vi "TelegramBOT_MainRPI.vi"() -> ()   [LabVIEW 2019]
uses:
  <vilib>/MakerHub/LINX/Private/Type Defs/LINX Ref.ctl
  <vilib>/MakerHub/LINX/Private/Type Defs/Platform.ctl
  <vilib>/MakerHub/LINX/Private/Type Defs/Interface.ctl
  <vilib>/MakerHub/LINX/Private/Device/Type Defs/LINX Device Config.ctl
  <vilib>/MakerHub/LINX/Private/Device/Type Defs/TCP Config.ctl
  <vilib>/MakerHub/LINX/Private/Device/Type Defs/Channels.ctl
  Demo 2 Sensor_SHT21/SHT21_class/SHT21.lvclass
  TelegramBOT_class/SendMsgType.ctl
  TelegramBOT_class/KeyboardMarkup.ctl
  <vilib>/MakerHub/LINX/Public/Peripherals/Digital/Digital Write 1 Chan.vi
  <vilib>/MakerHub/LINX/Public/Peripherals/Digital/Digital Write N Chans.vi
  <vilib>/MakerHub/LINX/Private/Local IO/LinxDigitalWrite.vi
  <vilib>/MakerHub/LINX/Public/Utilities/Check Channel.vi
  <vilib>/MakerHub/LINX/Private/Local IO/Handle Errors.vi
  <vilib>/MakerHub/LINX/Public/Utilities/Open Local.vi
  <vilib>/MakerHub/LINX/Private/Utilties/Generate Error.vi
  TelegramBOT_class/TelegramBOT.lvclass
  <vilib>/MakerHub/LINX/LMH-LINX.lvlib
  <vilib>/MakerHub/LINX/Private/Device/Device.lvlib
panel:
  out "From":string
  out "Message":string
  out "Message counter":i32
  in  "Stop":bool
  out "error out":errorcluster
  out "Connection":bool
  # "Demo live at our booth"
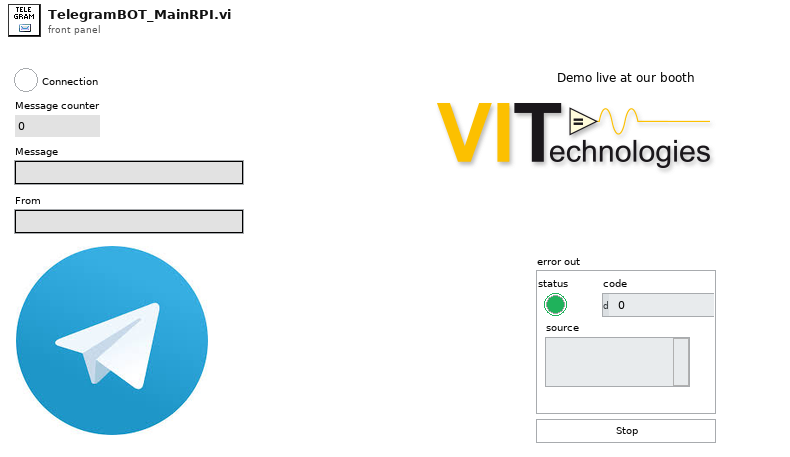
[diagram p1: front panel]
types:
  T1 = typedef "LMH-LINX.lvlib/LINX Ref.ctl" = cluster{"IO":T2, "Interface":T3, "LINX Device Config":T4}
  T2 = typedef "LMH-LINX.lvlib/Platform.ctl" = enum16{"Remote", "Local"}
  T3 = typedef "LMH-LINX.lvlib/Interface.ctl" = enum16{"Serial", "TCP"}
  T4 = typedef "LMH-LINX.lvlib/Device.lvlib/LINX Device Config.ctl" = cluster{"Interface":T3, "COM Port":refnum<visa-resource-name>, "TCP Configuration":T5, "Device Family":u8, "Device ID":u8, "Device Name":string, "TCP Ref":refnum<k5>, "Channels":T6}
  T5 = typedef "LMH-LINX.lvlib/Device.lvlib/TCP Config.ctl" = cluster{"IP Address":string, "Port":u16}
  T6 = typedef "LMH-LINX.lvlib/Channels.ctl" = cluster{"DI":u8[], "DO":u8[], "AI":u8[], "AO":u8[], "PWM":u8[], "QE":u8[], "UART":u8[], "I2C 2":u8[], "SPI":u8[], "CAN":u8[], "Servo":u8[], "AI Ref (V)":dbl, "AI Resolution (Bits)":u8, "AO Ref (V)":dbl, "AO Resolution (Bits)":u8}
  T7 = cluster{"LINX":T1, "SHT21":refnum<class "SHT21.lvclass">}
  T8 = typedef "TelegramBOT.lvclass/KeyboardMarkup.ctl" = cluster{"keyboard":cluster{"text":string, "req_loc":bool}[][], "resize_keyboard":bool, "one_time_keyboard":bool, "selective":bool}
  T9 = typedef "TelegramBOT.lvclass/SendMsgType.ctl" = enum16{"Text", "ReplyKeyboardMarkup", "ReplyKeyboardRemove"}
  T10 = typedef "TelegramBOT.lvclass/MessageCluster.ctl" = cluster{"update_id":u32, "from":string, "text":string, "date":timestamp, "chat_id":i32, "type":string, "reply_to_message.text":string, "message_id":u32}
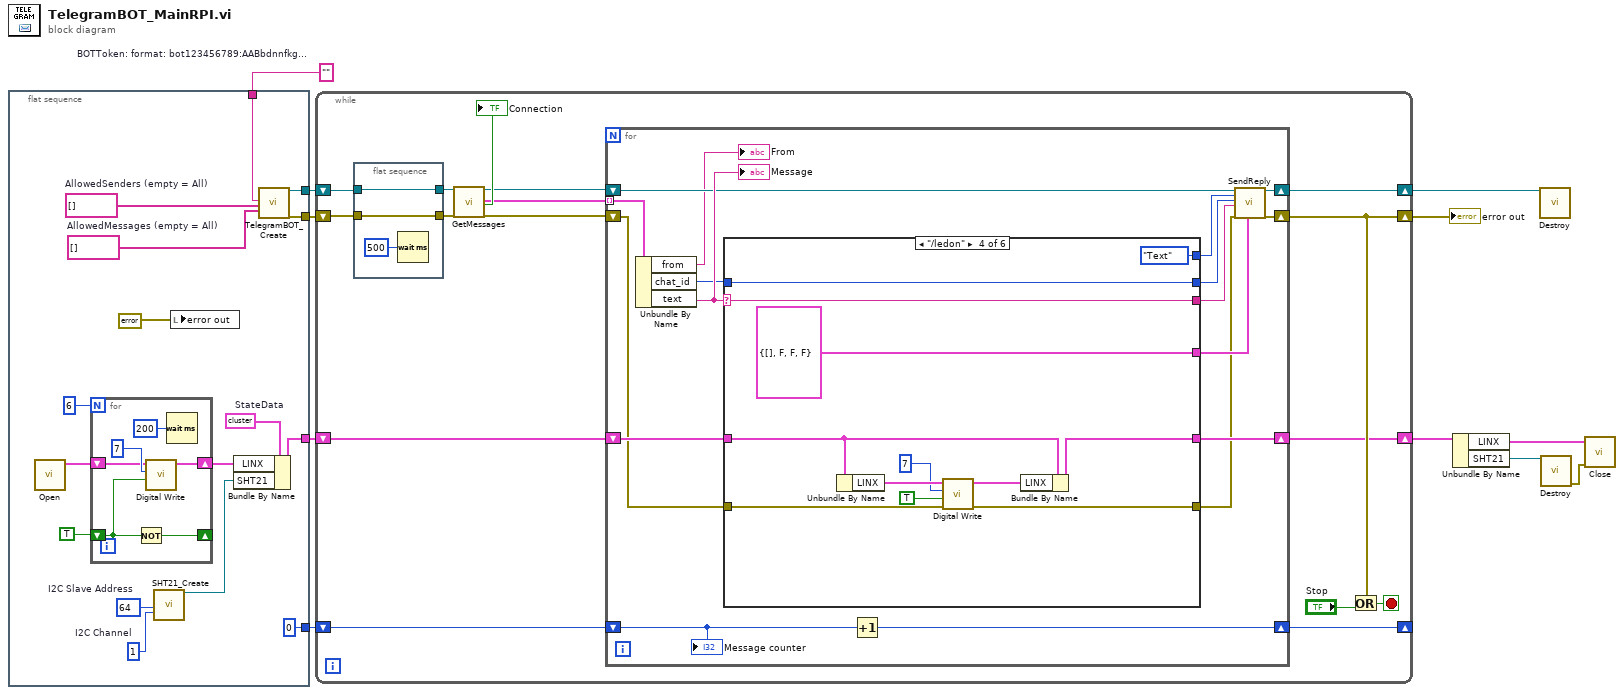
[diagram p0: block diagram]
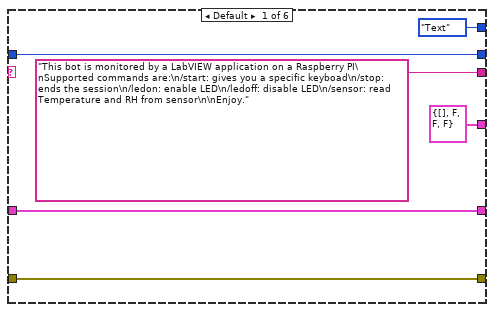
[diagram p2: hidden frame]
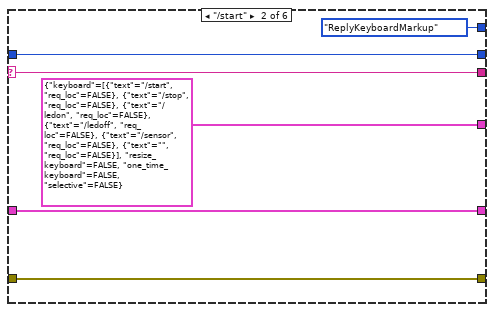
[diagram p3: hidden frame]
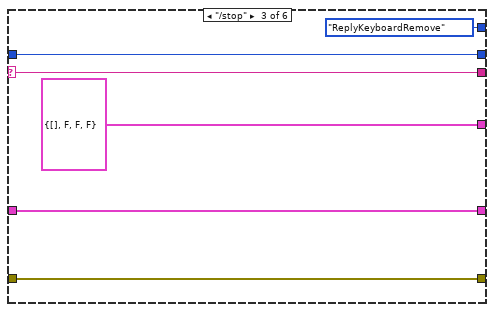
[diagram p4: hidden frame]
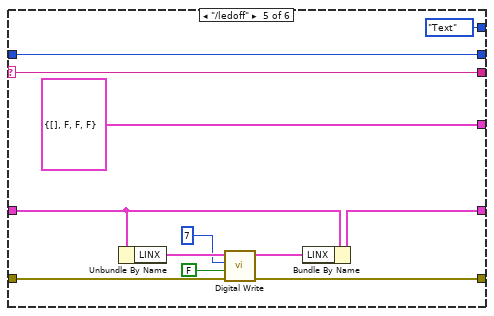
[diagram p5: hidden frame]
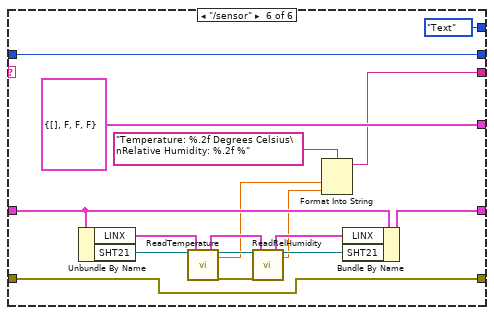
[diagram p6: hidden frame]
diagram:
  w7 = ""  # BOTToken: format: bot123456789:AABbdnnfkg...
  n1 = flat-sequence {
    tunnel: [w27] -> w11
    tunnel: [w26] -> w10
    tunnel: [0] -> w8
    tunnel: w7 -> [w24]
    tunnel: [w18] -> w1
    frame #0 {
      w20 = u8 1  # I2C Channel
      w21 = u8 64  # I2C Slave Address
      w19 = T7 {"LINX"={"IO"=enum."Remote", "Interface"=enum."Serial", "LINX Device Config"={"Interface"=enum."Serial", "COM Port"="COM13", "TCP Configuration"={"IP Address"="", "Port"=0}, "Device Family"=1, "Device ID"=1, "Device Name"="myRIO-1900", "TCP Ref"=refnum, "Channels"={"DI"=[0, 1, 2, 3, 4, 5, 6, 7, 8, 9, 10, 11, 12, 13, 14, 15, 16, 17, 18, 19, 20, 21, 22, 23, 24, 25, 26, 27, 28, 29, 30, 31, 32, 33, 34, 35, 36, 37, 38, 39, 40, 41, 42, 43, 44, 45, 46], "DO"=[0, 1, 2, 3, 4, 5, 6, 7, 8, 9, 10, 11, 12, 13, 14, 15, 16, 17, 18, 19, 20, 21, 22, 23, 24, 25, 26, 27, 28, 29, 30, 31, 32, 33, 34, 35, 36, 37, 38, 39, 40, 41, 42, 43, 44, 45, 46], "AI"=[0, 1, 2, 3, 4, 5, 6, 7, 8, 9, 10, 11], "AO"=[], "PWM"=[3, 5, 6, 9, 10], "QE"=[], "UART"=[0, 1], "I2C 2"=[0], "SPI"=[0], "CAN"=[], "Servo"=[], "AI Ref (V)"=0.0, "AI Resolution (Bits)"=0, "AO Ref (V)"=0.0, "AO Resolution (Bits)"=0}}}, "SHT21"=refnum}  # StateData
      w22 = string[] []  # AllowedMessages (empty = All)
      w23 = string[] []  # AllowedSenders (empty = All)
      n2 = call-poly <vilib>:"Open.vi"() -> ("LINX Resource"=w15:T1)  [unwired: 9 in, 2 out]
      n3 = for {
        N: 6 -> [_]
        shift-right: [w31] -> w14
        shift-left: w15 -> [w32]
        shift-right: [w30] -> _
        shift-left: TRUE ("Output Value") -> [w29]
        n4 = Not(x=w29) -> (.not. x?=w30:bool)
        n5 = call-poly <vilib>:"Digital Write.vi"("Output Value"=w29, "DO Channel"=u8 7, "LINX Resource"=w32) -> ("LINX Resource"=w31:T1)  [unwired: 7 in, 1 out]
        n6 = Wait (ms)(milliseconds to wait=u32 200) -> ()  [unwired: 1 out]
      }
      n7 = call "SHT21_Create.vi"("I2C Slave Address (0)"=w21, "I2C Channel (0)"=w20) -> ("reference out"=w17:refnum<class "SHT21.lvclass">)  [unwired: 16 in, 1 out]
      n8 = local write "error out"(errorcluster {"status"=FALSE, "code"=0, "source"=""} ("error out")) -> ()
      n9 = Bundle By Name(cluster=w19, "LINX"=w14, "SHT21"=w17) -> (w18:T7)
      n10 = call "TelegramBOT_Create.vi"("BOTToken(bot<token>)"=w24, "AllowedSenders (empty = All)"=w23, "AllowedMessages (empty = All)"=w22) -> ("reference out"=w27:refnum<class "TelegramBOT.lvclass">, "error out"=w26:errorcluster)  [unwired: 15 in]
    }
  }
  n11 = while {
    shift-right: [w34] -> w5
    shift-left: w1 -> [w35]
    shift-right: [w38] -> w6
    shift-left: w10 -> [w44]
    shift-right: [w42] -> w9
    shift-left: w11 -> [w45]
    shift-right: [w36] -> _
    shift-left: w8 -> [w37]
    stop <- w48 stop-if-true
    n12 = flat-sequence {
      tunnel: [w128] -> w46
      tunnel: w45 -> [w128]
      tunnel: [w127] -> w47
      tunnel: w44 -> [w127]
      frame #0 {
        n13 = Wait (ms)(milliseconds to wait=u32 500) -> ()  [unwired: 1 out]
      }
    }
    n14 = call-dynamic "GetMessages.vi"("reference in"=w46, "error in (no error)"=w47) -> ("reference out"=w41:refnum<class "TelegramBOT.lvclass">, "Messages"=w40:T10[], "Connection"=→"Connection":bool, "error out"=w39:errorcluster)  [unwired: 13 in, 1 out]
    n15 = for {
      shift-right: [w62] -> w42
      shift-left: w41 -> [w63]
      shift-right: [w61] -> w38
      shift-left: w39 -> [w51]
      tunnel: w40 -> [w66] mode=indexing
      shift-right: [w52] -> w34
      shift-left: w35 -> [w54]
      shift-right: [w55] -> w36
      shift-left: w37 -> [w56]
      n16 = Unbundle By Name(w66) -> ("from"=→"From":string, "chat_id"=w64:i32, "text"=w65:string)
      "Message" <- w65
      n17 = case shown="\"/ledon\"" w65 {
        selector: w65 -> [_ w78 w84 w96 w108 _]
        tunnel: w64 -> [w72 w77 w83 w95 w107 w125]
        tunnel: ["This bot is monitored by a LabVIEW application on a Raspberry PI\nSupported commands are:\n/start: gives you a specific keyboad\n/stop: ends the session\n/ledon: enable LED\n/ledoff: disable LED\n/sensor: read Temperature and RH from sensor\n\nEnjoy." w78 w84 w96 w108 w110] -> w60
        tunnel: [w72 w77 w83 w95 w107 w125] -> w59
        tunnel: [SendMsgType."Text" ("MsgType") SendMsgType."ReplyKeyboardMarkup" ("MsgType") SendMsgType."ReplyKeyboardRemove" ("MsgType") SendMsgType."Text" ("MsgType") SendMsgType."Text" ("MsgType") SendMsgType."Text" ("MsgType")] -> w58
        tunnel: [T8 {"keyboard"=[], "resize_keyboard"=FALSE, "one_time_keyboard"=FALSE, "selective"=FALSE} ("ReplyKeyboardMarkup") T8 {"keyboard"=[[{"text"="/start", "req_loc"=FALSE}, {"text"="/stop", "req_loc"=FALSE}], [{"text"="/ledon", "req_loc"=FALSE}, {"text"="/ledoff", "req_loc"=FALSE}], [{"text"="/sensor", "req_loc"=FALSE}, {"text"="", "req_loc"=FALSE}]], "resize_keyboard"=FALSE, "one_time_keyboard"=FALSE, "selective"=FALSE} ("ReplyKeyboardMarkup") T8 {"keyboard"=[], "resize_keyboard"=FALSE, "one_time_keyboard"=FALSE, "selective"=FALSE} ("ReplyKeyboardMarkup") T8 {"keyboard"=[], "resize_keyboard"=FALSE, "one_time_keyboard"=FALSE, "selective"=FALSE} ("ReplyKeyboardMarkup") T8 {"keyboard"=[], "resize_keyboard"=FALSE, "one_time_keyboard"=FALSE, "selective"=FALSE} ("ReplyKeyboardMarkup") T8 {"keyboard"=[], "resize_keyboard"=FALSE, "one_time_keyboard"=FALSE, "selective"=FALSE} ("ReplyKeyboardMarkup")] -> w57
        tunnel: w54 -> [w68 w74 w80 w92 w97 w117]
        tunnel: [w68 w74 w80 w87 w98 w118] -> w52
        tunnel: w51 -> [w67 w73 w79 w89 w100 w109]
        tunnel: [w67 w73 w79 w88 w99 w109] -> w50
        frame Default {
        }
        frame "/start" {
        }
        frame "/stop" {
        }
        frame "/ledon" {
          n18 = Unbundle By Name(w92) -> ("LINX"=w91:T1)
          n19 = call-poly <vilib>:"Digital Write.vi"("Error In"=w89, "Output Value"=TRUE, "DO Channel"=u8 7, "LINX Resource"=w91) -> ("Error Out"=w88:errorcluster, "LINX Resource"=w86:T1)  [unwired: 6 in]
          n20 = Bundle By Name(cluster=w92, "LINX"=w86) -> (w87:T7)
        }
        frame "/ledoff" {
          n21 = Unbundle By Name(w97) -> ("LINX"=w104:T1)
          n22 = call-poly <vilib>:"Digital Write.vi"("Error In"=w100, "Output Value"=FALSE, "DO Channel"=u8 7, "LINX Resource"=w104) -> ("Error Out"=w99:errorcluster, "LINX Resource"=w102:T1)  [unwired: 6 in]
          n23 = Bundle By Name(cluster=w97, "LINX"=w102) -> (w98:T7)
        }
        frame "/sensor" {
          n24 = Unbundle By Name(w117) -> ("LINX"=w119:T1, "SHT21"=w120:refnum<class "SHT21.lvclass">)
          n25 = call-dynamic "ReadTemperature.vi"("reference in"=w120, "LINX Resource"=w119) -> ("LINX Resource"=w115:T1, "reference out"=w121:refnum<class "SHT21.lvclass">, "Temperature"=w113:dbl, "error out"=w122:errorcluster)  [unwired: 13 in, 1 out]
          n26 = call-dynamic "ReadRelHumidity.vi"("reference in"=w121, "error in (no error)"=w122, "LINX Resource"=w115) -> ("LINX Resource"=w114:T1, "reference out"=w116:refnum<class "SHT21.lvclass">, "RH"=w112:dbl)  [unwired: 12 in, 2 out]
          n27 = Format Into String(format string="Temperature: %.2f Degrees Celsius\nRelative Humidity: %.2f %", w113, w112) -> (resulting string=w110:string)  [unwired: 2 in, 1 out]
          n28 = Bundle By Name(cluster=w117, "LINX"=w114, "SHT21"=w116) -> (w118:T7)
        }
      }
      n29 = Increment(x=w56) -> (x+1=w55:i32)
      n30 = call-dynamic "SendReply.vi"("reference in"=w63, "MsgType"=w58, "ChatId"=w59, "Text"=w60, "error in (no error)"=w50, "ReplyKeyboardMarkup"=w57) -> ("reference out"=w62:refnum<class "TelegramBOT.lvclass">, "error out"=w61:errorcluster)  [unwired: 12 in]
      "Message counter" <- w56
    }
    n31 = Or(x=w38, y="Stop") -> (x .or. y?=w48:bool)
  }
  "error out" <- w6
  n32 = Unbundle By Name(w5) -> ("LINX"=w4:T1, "SHT21"=w3:refnum<class "SHT21.lvclass">)
  n33 = call-dynamic "Destroy.vi"("reference in"=w9) -> ()  [unwired: 17 in, 2 out]
  n34 = call-dynamic "Destroy.vi"("reference in"=w3) -> ("error out"=w2:errorcluster)  [unwired: 17 in, 1 out]
  n35 = call <vilib>:"Close.vi"("Error In"=w2, "LINX Resource"=w4) -> ()  [unwired: 9 in, 1 out]
